vi "Calculate center.vi"(11 "array":dbl[][](array[numeric])) -> (3 "Tray Center":dbl[](array[numeric])=[472.8869567258022, 109.34055613080434, 59.0791979543358, 1.5763766432237363])   [LabVIEW 2016]
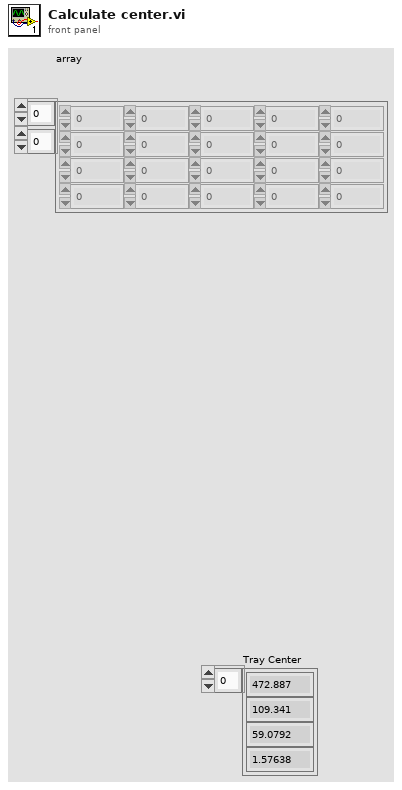
[diagram p1: front panel]
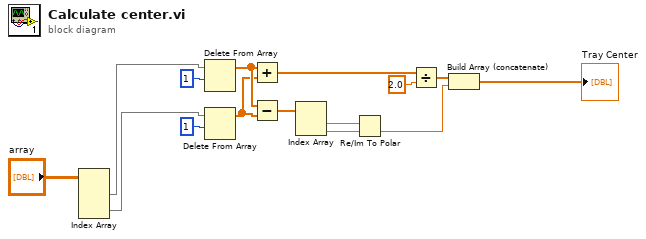
[diagram p0: block diagram]
diagram:
  n1 = Index Array(array="array") -> (element #1=w9:dbl[], element #2=w8:dbl[])  [unwired: 4 in]
  n2 = Delete From Array(array=w9, length=1) -> (array with subset deleted=w7:dbl[])  [unwired: 1 in, 1 out]
  n3 = Delete From Array(array=w8, length=1) -> (array with subset deleted=w6:dbl[])  [unwired: 1 in, 1 out]
  n4 = Add(x=w7, y=w6) -> (x+y=w14:dbl[])
  n5 = Subtract(x=w7, y=w6) -> (x-y=w5:dbl[])
  n6 = Index Array(array=w5) -> (element #1=w4:dbl, element #2=w3:dbl)  [unwired: 2 in]
  n7 = Re/Im To Polar(2:w3, 3:w4) -> (0:w2:dbl)  [unwired: 1 out]
  n8 = Divide(x=w14, y=2.0) -> (x/y=w15:dbl[])
  n9 = Build Array (concatenate)(w15, w2) -> (→"Tray Center":dbl[])
